vi "BrowseData.vi"(8 "ErrorIn(No Error)":errorcluster caption="entrée d'erreur (pas d'erreur)", 9 "MainProgQEvent":refnum<user-event>, 10 "MainProgQ":refnum<queue>, 11 "Interface en entrée":refnum<class "Interface.lvclass"> caption="DNL_LabVIEW Object in") -> (0 "sortie d'erreur":errorcluster, 3 "Interface en sortie":refnum<class "Interface.lvclass"> caption="DNL_LabVIEW Object out")   [LabVIEW 2019, in "Interface.lvclass"]
uses:
  Interface.lvclass
  BrowseDataStates.ctl
  ScanParams.ctl
  Interface.lvclass/Interface.ctl
panel:
  out "Header path":path
  out "Data path":path
  in  "YPar Sel":bool
  in  "Open2D":bool
  in  "Y Parameters":u16(ring) items=["AttoX.ReqPosition(um)", "AttoX.DetPos(um)", "AttoY.ReqPosition(um)", "AttoY.DetPos(um)", "MH150.Counts Ch1(ph)", "MH150.Counts Ch2(ph)", "MH150.Counts Chs Sum(ph)"]
  out "FilesPath":path[](array[path])
  out "Header String":string
  in  "CloseTreeStatus":bool
  in  "CloseTree":bool
  out "RangeString":string="??????"
  in  "Recheck Files":bool
  out "DateString":string="??????"
  in  "KeyWordFlt":bool
  in  "IncludeSubF":bool caption="Include SubFolders"
  in  "VarparFlt":bool
  in  "VarParam":string caption="Main Scan Parameter"
  in  "KeyWord":string
  in  "SessionFilt":bool
  in  "RangeFlt":bool
  in  "YearFlt":bool
  in  "DayFlt":bool
  in  "MonthFlt":bool
  in  "End Date":dbl=3629145600.0 format="%<%y/%m/%d>T"
  in  "Start Date":dbl format="%<%y/%m/%d>T"
  in  "Day":u8=1 min=1 max=31 step=1
  in  "Month":u8=1 min=1 max=12 step=1
  in  "Year":u16=2018 min=1960 max=2050 step=1
  in  "Session #":i32 min=0 max=1000 step=1
  out "VarPar":string
  out "CurveName":string
  in  "OpenCurve":bool
  in  "XPar Sel":bool
  in  "Data Folder Path":path
  in  "X Parameters":u16(ring) items=["AttoX.ReqPosition(um)", "AttoX.DetPos(um)", "AttoY.ReqPosition(um)", "AttoY.DetPos(um)", "MH150.Counts Ch1(ph)", "MH150.Counts Ch2(ph)", "MH150.Counts Chs Sum(ph)"]
  out "Curve Preview":cluster{"X Array":dbl[], "Y Array":dbl[]}(graph)
  out "DataPrev":string[][](array[string]) caption="File's Data Preview"
  in  "Arbre":string(tree)
  in  "stop":bool
  # "Filters"
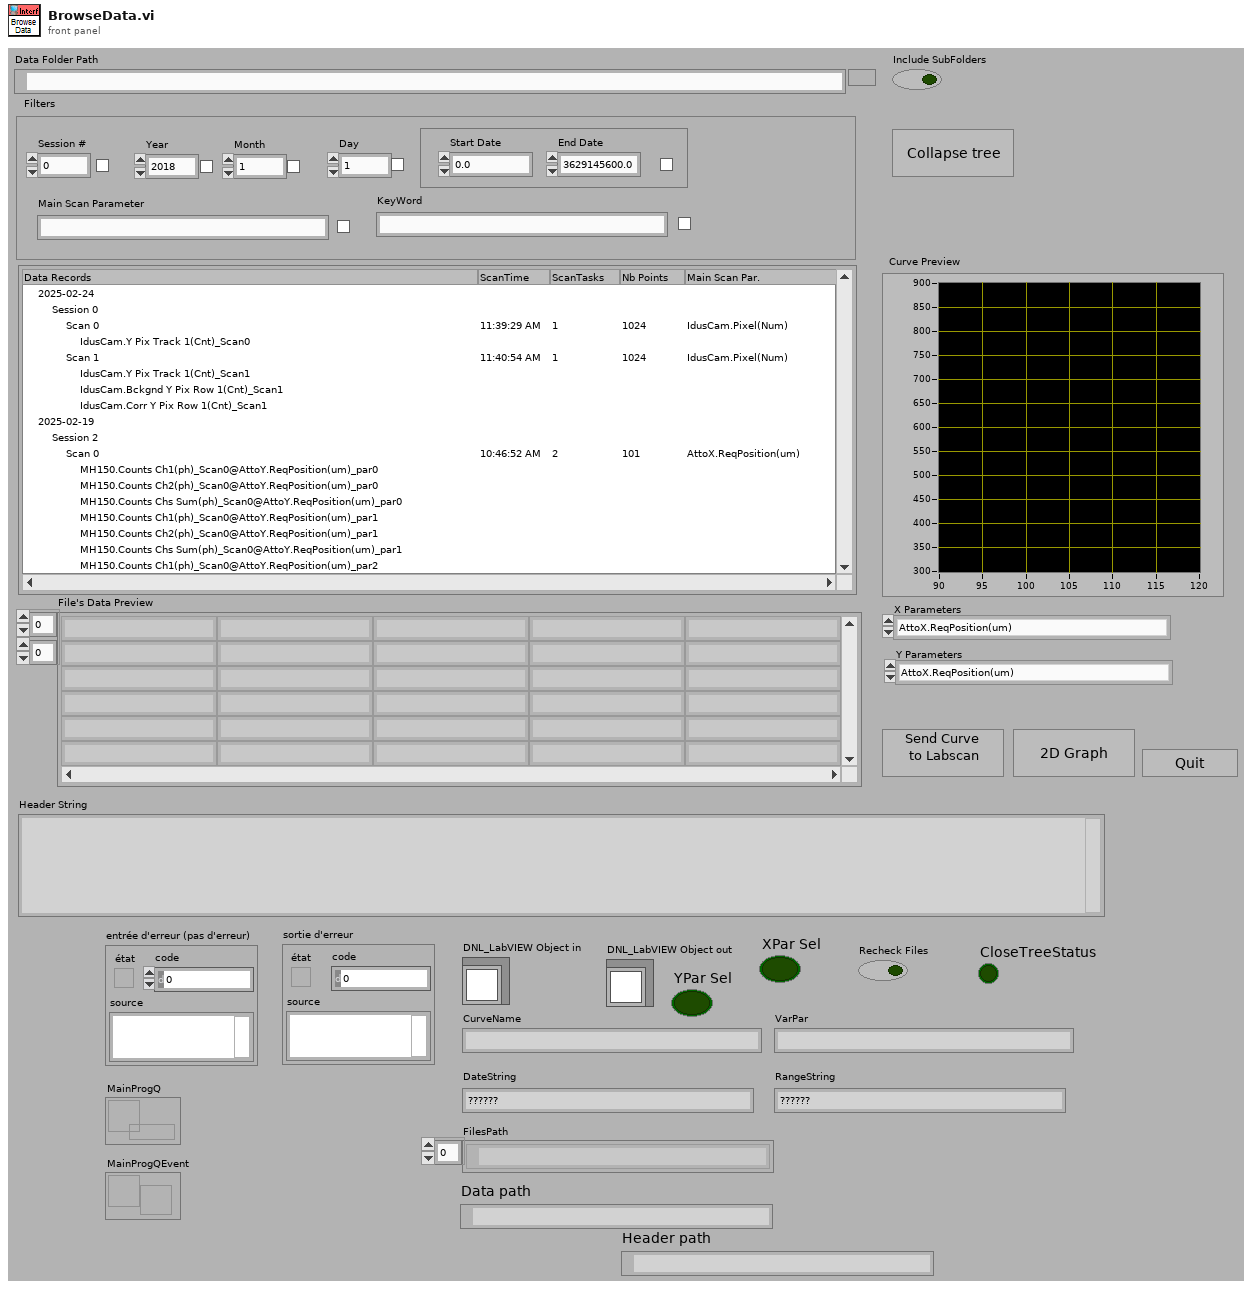
[diagram p1: front panel]
types:
  T1 = typedef "Interface.lvclass/ScanParams.ctl" = cluster{"Entête":string, "Scan list":string[], "NbCourbe":i32, "IndCourbe":i64, "NomDon":string[], "Session ":i32, "Date":string, "Time":string, "VarParams":string[][], "UserName":string, "ScanTableSize":i32[], "VarPar list":string[], "DescKeyword":string}
  T2 = typedef "BrowseDataStates.ctl" = enum16{"InitProg", "Delete File", "Opentxt", "LoadTree", "GetCurveData", "OpenCurve", "Open2D", "Stop"}
  T3 = enum8{"Enabled", "Disabled", "Disabled and Grayed Out"}
  T4 = enum16{"Enable", "Disable", "DisAndGrayed", "ReinitToDefVal", "EnumElementsArr"}
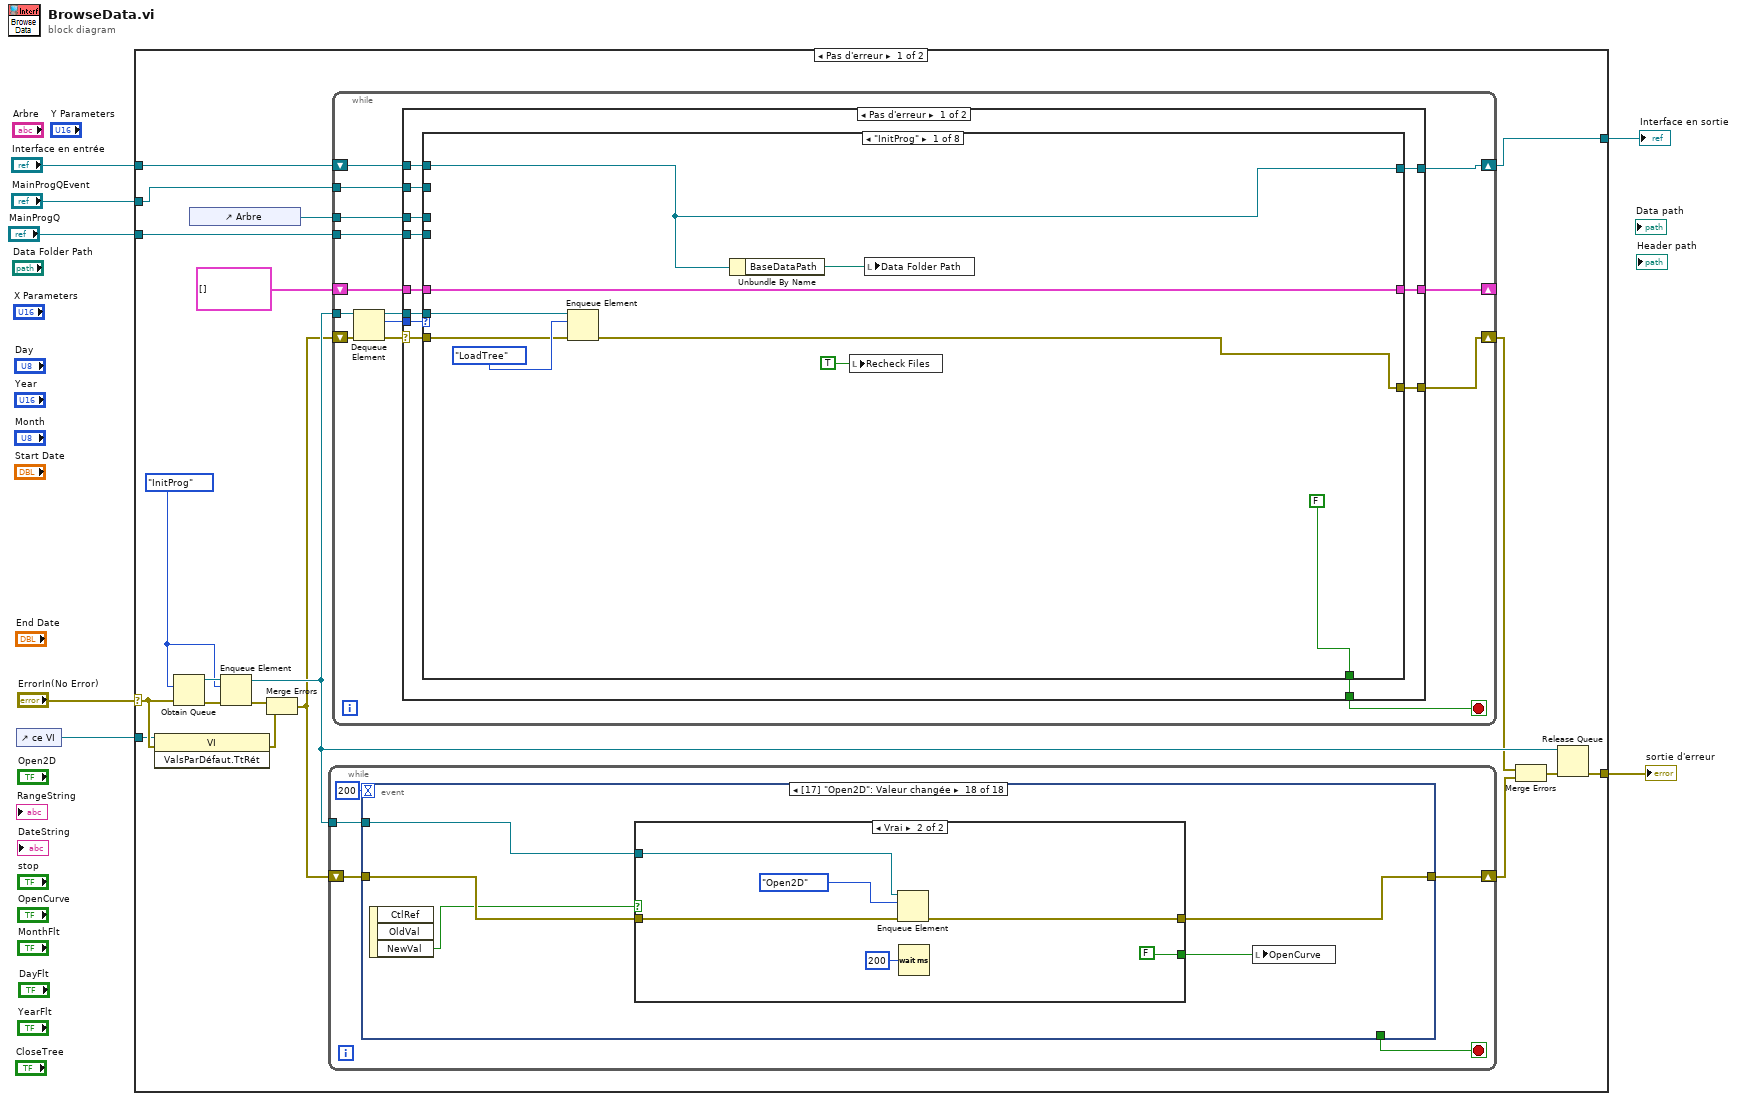
[diagram p0: block diagram]
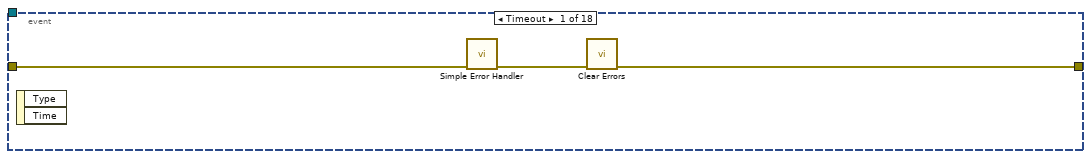
[diagram p2: hidden frame]
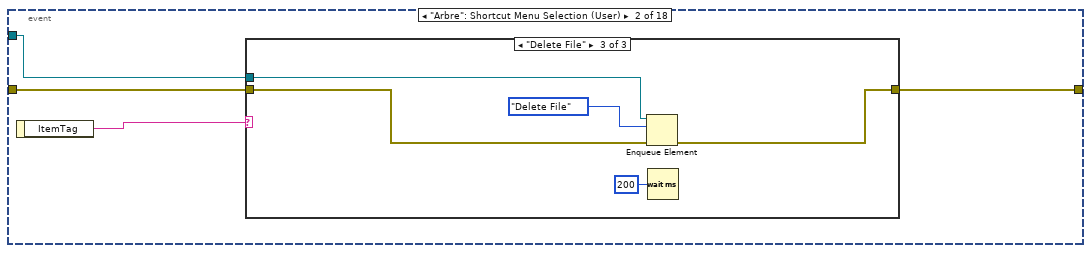
[diagram p3: hidden frame]
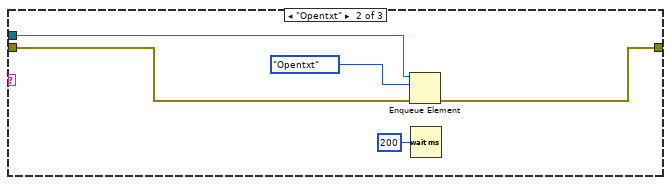
[diagram p5: hidden frame]
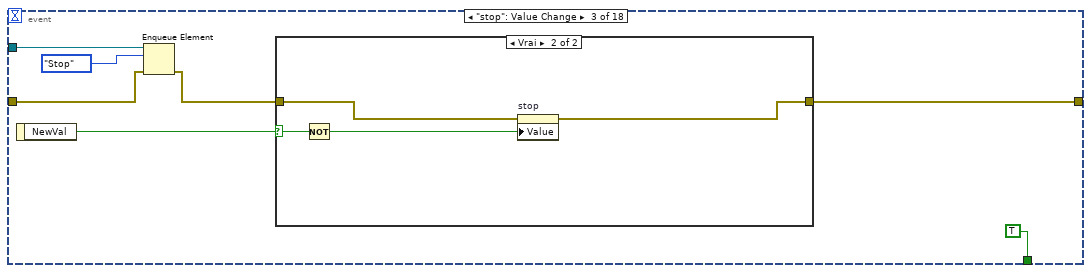
[diagram p6: hidden frame]
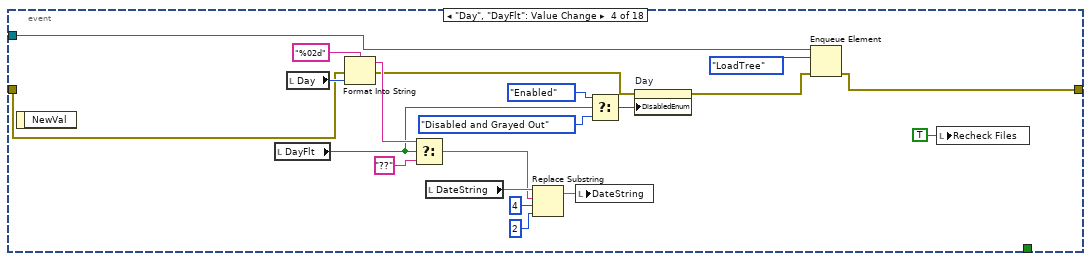
[diagram p8: hidden frame]
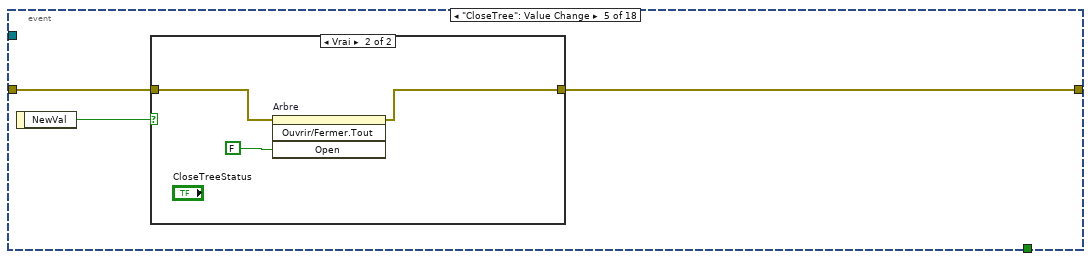
[diagram p9: hidden frame]
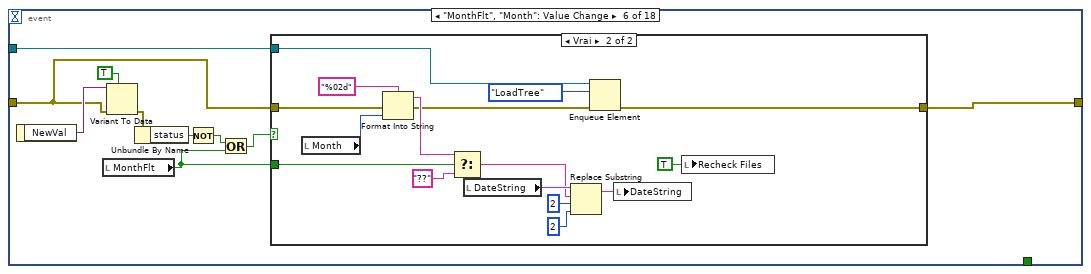
[diagram p11: hidden frame]
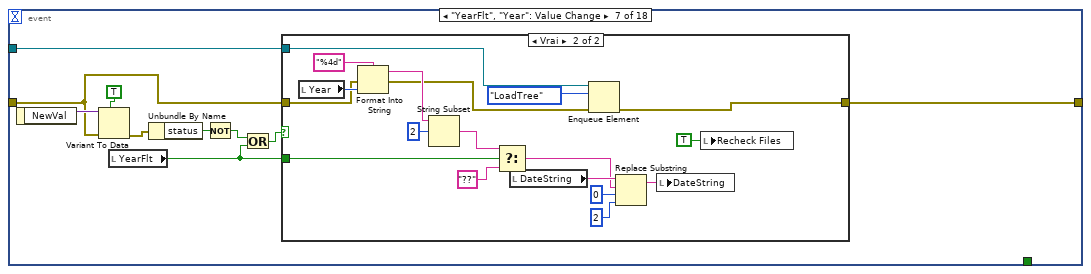
[diagram p13: hidden frame]
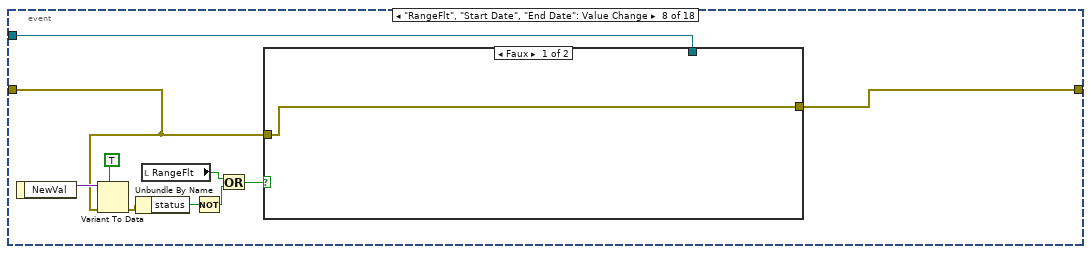
[diagram p15: hidden frame]
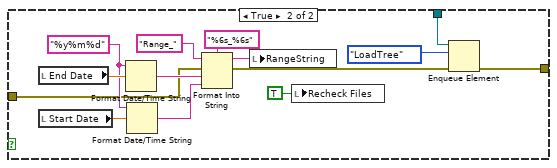
[diagram p16: hidden frame]
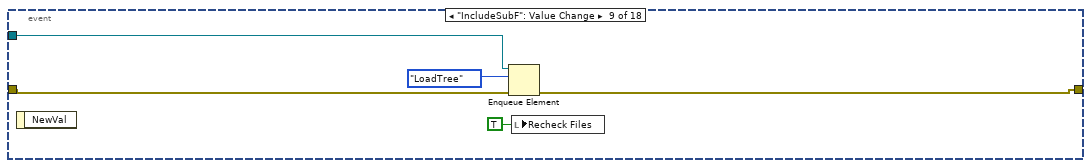
[diagram p17: hidden frame]
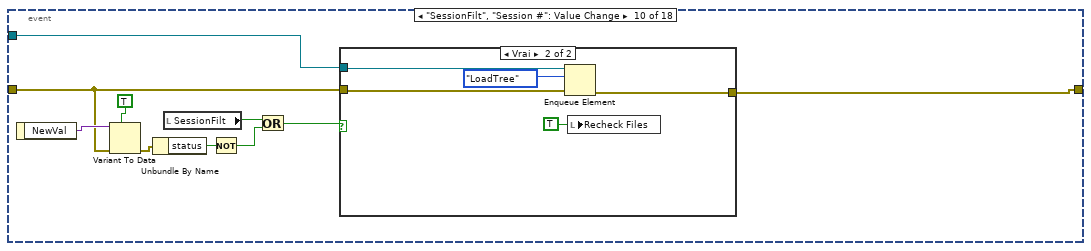
[diagram p18: hidden frame]
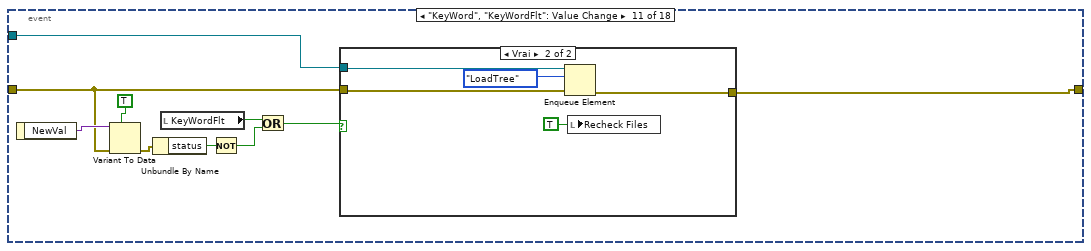
[diagram p20: hidden frame]
diagram:
  n1 = control-ref of="ce VI"() -> (w3:refnum<vi>)
  n2 = case shown="Pas d'erreur" "ErrorIn(No Error)" {
    selector: "ErrorIn(No Error)" -> [w13 w657]
    tunnel: [w23 w657] -> w6
    tunnel: "Interface en entrée" -> [w20 w656]
    tunnel: [w19 w656] -> w4
    tunnel: w3 -> [w12 _]
    tunnel: "MainProgQ" -> [w8 _]
    tunnel: "MainProgQEvent" -> [w9 _]
    frame No Error {
      w24 = BrowseDataStates."InitProg" ("Énum")
      n3 = invoke class="VI" method="ValsParDéfaut.TtRét"(reference=w12, error in=w13) -> (error out=w10:errorcluster)  [unwired: 1 in, 2 out]
      n4 = Obtain Queue(element data type=w24, error in (no error)=w13) -> (queue out=w25:refnum<queue>, error out=w26:errorcluster)  [unwired: 3 in, 1 out]
      n5 = control-ref of="Arbre"() -> (w18:refnum<vi>)
      n6 = Enqueue Element(queue=w25, element=w24, error in (no error)=w26) -> (queue out=w21:refnum<queue>, error out=w22:errorcluster)  [unwired: 1 in, 1 out]
      n7 = Merge Errors(w22, w10) -> (w11:errorcluster)
      n8 = while {
        shift-right: [w28] -> w15
        shift-left: w11 -> [w29]
        tunnel: w21 -> [w30]
        stop <- w27 stop-if-true
        n9 = event shown="[17] \"Open2D\": Valeur changée" {
          selector: _ -> [_ _ _ _ _ _ _ _ _ _ _ _ _ _ _ _ _ _]
          dyn-events: _ -> [_ _ _ _ _ _ _ _ _ _ _ _ _ _ _ _ _ _]
          timeout: 200 -> [_ _ _ _ _ _ _ _ _ _ _ _ _ _ _ _ _ _]
          tunnel: w30 -> [_ w35 w52 w63 _ w97 w124 w153 w170 w183 w199 w215 w224 w243 w256 _ w267 w280]
          tunnel: w29 -> [w34 w37 w54 w71 w83 w91 w121 w150 w172 w177 w193 w209 w229 w242 w253 w261 w266 w279]
          tunnel: [w32 w36 w55 w62 w82 w98 w125 w154 w171 w184 w200 w216 w225 w241 w257 w260 w268 w281] -> w28
          tunnel: [_ _ TRUE _ _ _ _ _ _ _ _ _ _ _ _ _ _ _] -> w27
          event Timeout {
            n10 = event-data() -> ()  [unwired: 1 in, 2 out]
            n11 = call <vilib>:"Simple Error Handler.vi"("error in (no error)"=w34) -> ("error out"=w33:errorcluster)  [unwired: 4 in, 4 out]
            n12 = call <vilib>:"Clear Errors.vi"("error in (no error)"=w33) -> ("error out"=w32:errorcluster)  [unwired: 5 in, 1 out]
          }
          event "Arbre": Shortcut Menu Selection (User) {
            n13 = event-data() -> ("ItemTag"=w38:string)  [unwired: 1 in]
            n14 = case shown="\"Delete File\"" w38 {
              tunnel: w37 -> [w39 w42 w47]
              tunnel: [w39 w41 w46] -> w36
              tunnel: w35 -> [_ w40 w45]
              frame Default {
              }
              frame "Opentxt" {
                n15 = Enqueue Element(queue=w40, element=BrowseDataStates."Opentxt" ("Énum"), error in (no error)=w42) -> (error out=w41:errorcluster)  [unwired: 1 in, 2 out]
                n16 = Wait (ms)(milliseconds to wait=u32 200 ("attente (ms)")) -> ()  [unwired: 1 out]
              }
              frame "Delete File" {
                n17 = Enqueue Element(queue=w45, element=BrowseDataStates."Delete File" ("Énum"), error in (no error)=w47) -> (error out=w46:errorcluster)  [unwired: 1 in, 2 out]
                n18 = Wait (ms)(milliseconds to wait=u32 200 ("attente (ms)")) -> ()  [unwired: 1 out]
              }
            }
          }
          event "stop": Value Change {
            n19 = event-data() -> ("NewVal"=w56:bool)  [unwired: 1 in]
            n20 = Enqueue Element(queue=w52, element=BrowseDataStates."Stop" ("Énum"), error in (no error)=w54) -> (error out=w53:errorcluster)  [unwired: 1 in, 2 out]
            n21 = case shown="Vrai" w56 {
              selector: w56 -> [_ w61]
              tunnel: w53 -> [w57 w59]
              tunnel: [w57 w58] -> w55
              frame False {
              }
              frame True {
                n22 = Not(x=w61) -> (.not. x?=w60:bool)
                n23 = property on="stop" class="Bool (strict)"(error in=w59, "Value"=w60) -> (error out=w58:errorcluster)  [unwired: 1 in, 1 out]
              }
            }
          }
          event "Day", "DayFlt": Value Change {
            n24 = event-data() -> ()  [unwired: 1 in, 1 out]
            n25 = local read "DayFlt"() -> (w70:bool)
            n26 = local read "Day"() -> (w79:u8)
            n27 = Format Into String(format string="%02d" ("chaîne de format"), error in=w71, w79) -> (resulting string=w74:string, error out=w67:errorcluster)  [unwired: 1 in]
            n28 = Select(t=w74, s=w70, f="??" ("cas faux")) -> (s? t:f=w73:string)
            n29 = local read "DateString"() -> (w80:string)
            n30 = Replace Substring(2:2 ("longueur (long. de la sous-chaîne)"), 3:4 ("offset (0)"), 4:w73, 5:w80) -> (1:w75:string)  [unwired: 1 out]
            n31 = local write "DateString"(w75) -> ()
            n32 = Select(t=T3."Enabled" ("Désactivé"), s=w70, f=T3."Disabled and Grayed Out" ("Désactivé")) -> (s? t:f=w66:T3)
            n33 = property on="Day" class="NumNb (strict)"(error in=w67, "DisabledEnum"=w66) -> (error out=w64:errorcluster)  [unwired: 1 in, 1 out]
            n34 = Enqueue Element(queue=w63, element=BrowseDataStates."LoadTree" ("Énum"), error in (no error)=w64) -> (error out=w62:errorcluster)  [unwired: 1 in, 2 out]
            n35 = local write "Recheck Files"(TRUE ("Recheck Files")) -> ()
          }
          event "CloseTree": Value Change {
            n36 = event-data() -> ("NewVal"=w84:bool)  [unwired: 1 in]
            n37 = case shown="Vrai" w84 {
              tunnel: w83 -> [w85 w88]
              tunnel: [w85 w87] -> w82
              frame False {
              }
              frame True {
                n38 = invoke on="Arbre" class="Arbre (strict)" method="Ouvrir/Fermer.Tout"(error in=w88, "Open"=FALSE ("Ouvrir ?")) -> (error out=w87:errorcluster)  [unwired: 2 in, 3 out]
              }
            }
          }
          event "MonthFlt", "Month": Value Change {
            n39 = event-data() -> ("NewVal"=w95:variant)  [unwired: 1 in]
            n40 = local read "MonthFlt"() -> (w89:bool)
            n41 = Variant To Data(error in=w91, type=TRUE, Variant=w95) -> (error out=w90:errorcluster)  [unwired: 1 out]
            n42 = Unbundle By Name(w90) -> ("status"=w94:bool)
            n43 = Not(x=w94) -> (.not. x?=w93:bool)
            n44 = Or(x=w93, y=w89) -> (x .or. y?=w92:bool)
            n45 = case shown="Vrai" w92 {
              tunnel: [w99 w104] -> w98
              tunnel: w97 -> [_ w103]
              tunnel: w91 -> [w99 w102]
              tunnel: w89 -> [_ w101]
              frame False {
              }
              frame True {
                n46 = local read "Month"() -> (w113:u8)
                n47 = Format Into String(format string="%02d" ("chaîne de format"), error in=w102, w113) -> (resulting string=w108:string, error out=w100:errorcluster)  [unwired: 1 in]
                n48 = Select(t=w108, s=w101, f="??" ("cas faux")) -> (s? t:f=w107:string)
                n49 = local read "DateString"() -> (w114:string)
                n50 = Replace Substring(2:2 ("longueur (long. de la sous-chaîne)"), 3:2 ("offset (0)"), 4:w107, 5:w114) -> (1:w109:string)  [unwired: 1 out]
                n51 = Enqueue Element(queue=w103, element=BrowseDataStates."LoadTree" ("Énum"), error in (no error)=w100) -> (error out=w104:errorcluster)  [unwired: 1 in, 2 out]
                n52 = local write "DateString"(w109) -> ()
                n53 = local write "Recheck Files"(TRUE ("Recheck Files")) -> ()
              }
            }
          }
          event "YearFlt", "Year": Value Change {
            n54 = event-data() -> ("NewVal"=w123:variant)  [unwired: 1 in]
            n55 = Variant To Data(error in=w121, type=TRUE, Variant=w123) -> (error out=w120:errorcluster)  [unwired: 1 out]
            n56 = local read "YearFlt"() -> (w116:bool)
            n57 = Unbundle By Name(w120) -> ("status"=w119:bool)
            n58 = Not(x=w119) -> (.not. x?=w117:bool)
            n59 = Or(x=w117, y=w116) -> (x .or. y?=w118:bool)
            n60 = case shown="Vrai" w118 {
              tunnel: w121 -> [w126 w135]
              tunnel: w116 -> [_ w134]
              tunnel: [w126 w132] -> w125
              tunnel: w124 -> [_ w131]
              frame False {
              }
              frame True {
                n61 = local read "Year"() -> (w142:u16)
                n62 = Format Into String(format string="%4d" ("chaîne de format"), error in=w135, w142) -> (resulting string=w130:string, error out=w127:errorcluster)  [unwired: 1 in]
                n63 = String Subset(string=w130, offset (0)=2) -> (substring=w128:string)  [unwired: 1 in]
                n64 = Select(t=w128, s=w134, f="??" ("cas faux")) -> (s? t:f=w137:string)
                n65 = local read "DateString"() -> (w143:string)
                n66 = Enqueue Element(queue=w131, element=BrowseDataStates."LoadTree" ("Énum"), error in (no error)=w127) -> (error out=w132:errorcluster)  [unwired: 1 in, 2 out]
                n67 = Replace Substring(2:2 ("longueur (long. de la sous-chaîne)"), 3:0 ("offset (0)"), 4:w137, 5:w143) -> (1:w138:string)  [unwired: 1 out]
                n68 = local write "DateString"(w138) -> ()
                n69 = local write "Recheck Files"(TRUE ("Recheck Files")) -> ()
              }
            }
          }
          event "RangeFlt", "Start Date", "End Date": Value Change {
            n70 = event-data() -> ("NewVal"=w152:variant)  [unwired: 1 in]
            n71 = Variant To Data(error in=w150, type=TRUE, Variant=w152) -> (error out=w149:errorcluster)  [unwired: 1 out]
            n72 = Unbundle By Name(w149) -> ("status"=w148:bool)
            n73 = local read "RangeFlt"() -> (w146:bool)
            n74 = Not(x=w148) -> (.not. x?=w147:bool)
            n75 = Or(x=w146, y=w147) -> (x .or. y?=w145:bool)
            n76 = case shown="Faux" w145 {
              tunnel: [w155 w166] -> w154
              tunnel: w153 -> [_ w165]
              tunnel: w150 -> [w155 w156]
              frame False {
              }
              frame True {
                w162 = "%y%m%d" ("chaîne de format de l'heure (%c)")
                n77 = local read "End Date"() -> (w164:dbl)
                n78 = local read "Start Date"() -> (w163:dbl)
                n79 = Format Date/Time String(time format string (%c)=w162, seconds (now)=w164) -> (date/time string=w160:string)  [unwired: 1 in]
                n80 = Format Date/Time String(time format string (%c)=w162, seconds (now)=w163) -> (date/time string=w161:string)  [unwired: 1 in]
                n81 = Format Into String(format string="%6s_%6s" ("chaîne de format"), initial string="Range_" ("chaîne initiale"), error in=w156, w160, w161) -> (resulting string=w158:string, error out=w157:errorcluster)
                n82 = local write "RangeString"(w158) -> ()
                n83 = local write "Recheck Files"(TRUE ("Recheck Files")) -> ()
                n84 = Enqueue Element(queue=w165, element=BrowseDataStates."LoadTree" ("Énum"), error in (no error)=w157) -> (error out=w166:errorcluster)  [unwired: 1 in, 2 out]
              }
            }
          }
          event "IncludeSubF": Value Change {
            n85 = event-data() -> ()  [unwired: 1 in, 1 out]
            n86 = Enqueue Element(queue=w170, element=BrowseDataStates."LoadTree" ("Énum"), error in (no error)=w172) -> (error out=w171:errorcluster)  [unwired: 1 in, 2 out]
            n87 = local write "Recheck Files"(TRUE ("Recheck Files")) -> ()
          }
          event "SessionFilt", "Session #": Value Change {
            n88 = event-data() -> ("NewVal"=w178:variant)  [unwired: 1 in]
            n89 = Variant To Data(error in=w177, type=TRUE, Variant=w178) -> (error out=w181:errorcluster)  [unwired: 1 out]
            n90 = Unbundle By Name(w181) -> ("status"=w180:bool)
            n91 = local read "SessionFilt"() -> (w175:bool)
            n92 = Not(x=w180) -> (.not. x?=w179:bool)
            n93 = Or(x=w175, y=w179) -> (x .or. y?=w176:bool)
            n94 = case shown="Vrai" w176 {
              tunnel: [w185 w188] -> w184
              tunnel: w183 -> [_ w187]
              tunnel: w177 -> [w185 w186]
              frame False {
              }
              frame True {
                n95 = Enqueue Element(queue=w187, element=BrowseDataStates."LoadTree" ("Énum"), error in (no error)=w186) -> (error out=w188:errorcluster)  [unwired: 1 in, 2 out]
                n96 = local write "Recheck Files"(TRUE ("Recheck Files")) -> ()
              }
            }
          }
          event "KeyWord", "KeyWordFlt": Value Change {
            n97 = event-data() -> ("NewVal"=w194:variant)  [unwired: 1 in]
            n98 = Variant To Data(error in=w193, type=TRUE, Variant=w194) -> (error out=w197:errorcluster)  [unwired: 1 out]
            n99 = Unbundle By Name(w197) -> ("status"=w196:bool)
            n100 = local read "KeyWordFlt"() -> (w191:bool)
            n101 = Not(x=w196) -> (.not. x?=w195:bool)
            n102 = Or(x=w191, y=w195) -> (x .or. y?=w192:bool)
            n103 = case shown="Vrai" w192 {
              tunnel: [w201 w204] -> w200
              tunnel: w199 -> [_ w203]
              tunnel: w193 -> [w201 w202]
              frame False {
              }
              frame True {
                n104 = Enqueue Element(queue=w203, element=BrowseDataStates."LoadTree" ("Énum"), error in (no error)=w202) -> (error out=w204:errorcluster)  [unwired: 1 in, 2 out]
                n105 = local write "Recheck Files"(TRUE ("Recheck Files")) -> ()
              }
            }
          }
          event "VarparFlt", "VarParam": Value Change {
            n106 = event-data() -> ("NewVal"=w210:variant)  [unwired: 1 in]
            n107 = Variant To Data(error in=w209, type=TRUE, Variant=w210) -> (error out=w213:errorcluster)  [unwired: 1 out]
            n108 = Unbundle By Name(w213) -> ("status"=w212:bool)
            n109 = local read "VarparFlt"() -> (w207:bool)
            n110 = Not(x=w212) -> (.not. x?=w211:bool)
            n111 = Or(x=w207, y=w211) -> (x .or. y?=w208:bool)
            n112 = case shown="Vrai" w208 {
              tunnel: [w217 w220] -> w216
              tunnel: w215 -> [_ w219]
              tunnel: w209 -> [w217 w218]
              frame False {
              }
              frame True {
                n113 = Enqueue Element(queue=w219, element=BrowseDataStates."LoadTree" ("Énum"), error in (no error)=w218) -> (error out=w220:errorcluster)  [unwired: 1 in, 2 out]
                n114 = local write "Recheck Files"(TRUE ("Recheck Files")) -> ()
              }
            }
          }
          event "Arbre": Value Change {
            n115 = event-data() -> ("CtlRef"=w231:refnum<vi>, "NewVal"=w230:string)  [unwired: 1 in]
            n116 = property class="Arbre (strict)"(reference=w231, error in=w229, "Active Item Tag"=w230) -> (error out=w226:errorcluster, "Indent Level"=w223:i32)  [unwired: 1 out]
            n117 = Equal?(x=w223, y=3 ("x")) -> (x = y?=w227:bool)
            n118 = case shown="Vrai" w227 {
              tunnel: w226 -> [w232 w240]
              tunnel: [w232 w239] -> w225
              tunnel: w224 -> [_ w238]
              tunnel: w223 -> [w235 _]
              frame False {
                n119 = Equal?(x=w235, y=2) -> (x = y?=w233:bool)
                n120 = case shown="Vrai" w233 {
                  frame False {
                  }
                  frame True {
                  }
                }
              }
              frame True {
                w236 = FALSE ("XPar Sel")
                n121 = local write "XPar Sel"(w236) -> ()
                n122 = local write "YPar Sel"(w236) -> ()
                n123 = Enqueue Element(queue=w238, element=BrowseDataStates."GetCurveData" ("Énum"), error in (no error)=w240) -> (error out=w239:errorcluster)  [unwired: 1 in, 2 out]
              }
            }
          }
          event "Data Folder Path": Value Change {
            n124 = event-data() -> ("OldVal"=w246:path, "NewVal"=w245:path)  [unwired: 1 in, 1 out]
            n125 = Not Equal?(x=w246, y=w245) -> (x != y?=w244:bool)
            n126 = case shown="Vrai" w244 {
              tunnel: w243 -> [_ w251]
              tunnel: w242 -> [w247 w250]
              tunnel: [w247 w249] -> w241
              frame False {
              }
              frame True {
                n127 = Enqueue Element(queue=w251, element=BrowseDataStates."LoadTree" ("Énum"), error in (no error)=w250) -> (error out=w249:errorcluster)  [unwired: 1 in, 2 out]
                n128 = local write "Recheck Files"(TRUE ("Recheck Files")) -> ()
              }
            }
          }
          event "X Parameters": Value Change {
            n129 = event-data() -> ()  [unwired: 1 in, 3 out]
            n130 = flat-sequence {
              tunnel: [w258] -> w254
              tunnel: w253 -> [w258]
              frame #0 {
                n131 = local write "XPar Sel"(TRUE ("XPar Sel")) -> ()
              }
            }
            n132 = Enqueue Element(queue=w256, element=BrowseDataStates."GetCurveData" ("Énum"), error in (no error)=w254) -> (error out=w257:errorcluster)  [unwired: 1 in, 2 out]
          }
          event "Y Parameters": Value Change {
            n133 = event-data() -> ()  [unwired: 1 in, 3 out]
            n134 = flat-sequence {
              tunnel: [w262] -> w260
              tunnel: w261 -> [w262]
              frame #0 {
                n135 = local write "YPar Sel"(TRUE ("XPar Sel")) -> ()
              }
            }
          }
          event "OpenCurve": Value Change {
            n136 = event-data() -> ("NewVal"=w265:bool)  [unwired: 1 in, 2 out]
            n137 = case shown="Vrai" w265 {
              tunnel: [w269 w276] -> w268
              tunnel: w267 -> [_ w275]
              tunnel: w266 -> [w269 w274]
              tunnel: [FALSE ("OpenCurve") FALSE ("OpenCurve")] -> w264
              frame False {
              }
              frame True {
                n138 = Enqueue Element(queue=w275, element=BrowseDataStates."OpenCurve" ("Énum"), error in (no error)=w274) -> (error out=w276:errorcluster)  [unwired: 1 in, 2 out]
                n139 = Wait (ms)(milliseconds to wait=u32 200 ("attente (ms)")) -> ()  [unwired: 1 out]
              }
            }
            n140 = local write "OpenCurve"(w264) -> ()
          }
          event "Open2D": Value Change {
            n141 = event-data() -> ("NewVal"=w278:bool)  [unwired: 1 in, 2 out]
            n142 = case shown="Vrai" w278 {
              tunnel: [w282 w289] -> w281
              tunnel: w280 -> [_ w288]
              tunnel: w279 -> [w282 w287]
              tunnel: [FALSE ("OpenCurve") FALSE ("OpenCurve")] -> w277
              frame False {
              }
              frame True {
                n143 = Enqueue Element(queue=w288, element=BrowseDataStates."Open2D" ("Énum"), error in (no error)=w287) -> (error out=w289:errorcluster)  [unwired: 1 in, 2 out]
                n144 = Wait (ms)(milliseconds to wait=u32 200 ("attente (ms)")) -> ()  [unwired: 1 out]
              }
            }
            n145 = local write "OpenCurve"(w277) -> ()
          }
        }
      }
      n146 = while {
        tunnel: w21 -> [w301]
        shift-right: [w297] -> w16
        shift-left: w11 -> [w299]
        shift-right: [w296] -> w19
        shift-left: w20 -> [w295]
        tunnel: w18 -> [w294]
        shift-right: [w293] -> _
        shift-left: T1[] [] ("Headers") -> [w292]
        tunnel: w9 -> [w291]
        tunnel: w8 -> [w290]
        stop <- w298 stop-if-true
        n147 = Dequeue Element(queue=w301, error in (no error)=w299) -> (queue out=w300:refnum<queue>, element=w302:T2, error out=w303:errorcluster)  [unwired: 1 in, 1 out]
        n148 = case shown="Pas d'erreur" w303 {
          selector: w303 -> [w313 w654]
          tunnel: w302 -> [w315 _]
          tunnel: w300 -> [w314 _]
          tunnel: [w312 FALSE] -> w298
          tunnel: [w311 w651] -> w297
          tunnel: [w310 w653] -> w296
          tunnel: w295 -> [w309 w653]
          tunnel: w294 -> [w308 _]
          tunnel: [w307 w652] -> w293
          tunnel: w292 -> [w306 w652]
          tunnel: w291 -> [w305 _]
          tunnel: w290 -> [w304 _]
          frame No Error {
            n149 = case shown="\"InitProg\"" w315 {
              tunnel: w314 -> [w321 _ _ _ w523 _ _ _]
              tunnel: w313 -> [w318 w337 w394 w500 w550 w597 w639 w649]
              tunnel: [FALSE FALSE _ _ _ _ _ TRUE] -> w312
              tunnel: [w316 w330 w390 w475 w524 w582 w609 w649] -> w311
              tunnel: [w323 w360 w385 w496 w546 w584 w641 w647] -> w310
              tunnel: w309 -> [w323 w360 w385 w496 w546 w598 w642 w647]
              tunnel: w308 -> [_ w359 w395 w501 w551 _ _ _]
              tunnel: [w319 w358 w387 w497 w547 w596 w646 w648] -> w307
              tunnel: w306 -> [w319 w343 w387 w497 w547 w596 w646 w648]
              tunnel: w305 -> [_ _ _ _ _ w586 _ _]
              tunnel: w304 -> [_ _ _ _ _ w585 _ _]
              frame "InitProg" {
                n150 = Enqueue Element(queue=w321, element=BrowseDataStates."LoadTree" ("Énum"), error in (no error)=w318) -> (error out=w316:errorcluster)  [unwired: 1 in, 2 out]
                n151 = Unbundle By Name(w323) -> ("BaseDataPath"=w322:path)
                n152 = local write "Recheck Files"(TRUE ("Recheck Files")) -> ()
                n153 = local write "Data Folder Path"(w322) -> ()
              }
              frame "LoadTree" {
                n154 = control-ref of="This VI"() -> (w336:refnum<vi>)
                n155 = property class="VI"(reference=w336, error in=w337) -> (error out=w335:errorcluster, "Panel"=w334:refnum<vi>)  [unwired: 1 out]
                n156 = property class="FA"(reference=w334, error in=w335, "DeferPanUpdts"=TRUE ("Defer Panel Updates")) -> (reference out=w333:refnum<vi>, error out=w328:errorcluster)
                n157 = local read "RangeString"() -> (w339:string)
                n158 = local read "DateString"() -> (w340:string)
                n159 = Select(t="Session #", s="SessionFilt", f=-1 ("cas faux")) -> (s? t:f=w344:i32)
                n160 = Select(t="VarParam", s="VarparFlt", f="" ("cas faux")) -> (s? t:f=w348:string)
                n161 = call <vilib>:"Set Busy.vi"("error in (no error)"=w328) -> ("error out"=w327:errorcluster)  [unwired: 9 in, 1 out]
                n162 = local read "Data Folder Path"() -> (w357:path)
                n163 = Select(t="KeyWord", s="KeyWordFlt", f="" ("cas faux")) -> (s? t:f=w352:string)
                n164 = Select(t=w339, s="RangeFlt", f=w340) -> (s? t:f=w338:string)
                n165 = call "DataTree_LS1.vi"("Arbre"=w359, "Data Folder Path"=w357, "ScanParamsIn"=w343, "VarParam"=w348, "Date String"=w338, "Session"=w344, "error in (no err)"=w327, "IncludeSubF"="IncludeSubF", "Recheck Files"="Recheck Files", "KeyWord"=w352) -> ("Headers Out"=w358:T1[], "FilesPath"=→"FilesPath":path[], "error out"=w326:errorcluster)  [unwired: 1 in, 2 out]
                n166 = call <vilib>:"Unset Busy.vi"("error in (no error)"=w326) -> ("error out"=w325:errorcluster)  [unwired: 10 in]
                n167 = property class="FA"(reference=w333, error in=w325, "DeferPanUpdts"=FALSE ("Defer Panel Updates")) -> (error out=w330:errorcluster)  [unwired: 1 out]
              }
              frame "GetCurveData" {
                n168 = property class="Arbre (strict)"(reference=w395, error in=w394) -> (error out=w379:errorcluster, "Active Item Tag"=w378:string)  [unwired: 1 out]
                n169 = Scan From String(format string="%4s-%2s-%2s_S%d_Sc%d_%d_f%d" ("chaîne de format"), input string=w378, error in=w379, default 5=i64 0 ("valeur par défaut 5")) -> (error out=w380:errorcluster, output 6=w381:i32, output 7=w383:i32)  [unwired: 12 in, 2 out]
                n170 = case shown="Pas d'erreur" w380 {
                  selector: w380 -> [w396 _]
                  tunnel: w383 -> [w398 _]
                  tunnel: [w398 w400] -> w363
                  tunnel: [w397 w399] -> w382
                  tunnel: w381 -> [w397 _]
                  tunnel: [w396 w401] -> w372
                  tunnel: w379 -> [_ w402]
                  tunnel: w378 -> [_ w405]
                  tunnel: "%4s-%2s-%2s_S%d_Sc%d_%d_%d_f%d" ("chaîne de format") -> [_ w404]
                  frame No Error {
                  }
                  frame Error {
                    n171 = Scan From String(format string=w404, input string=w405, error in=w402, default 5=i64 0 ("valeur par défaut 5")) -> (error out=w401:errorcluster, output 7=w399:i32, output 8=w400:i32)  [unwired: 14 in, 2 out]
                  }
                }
                n172 = local read "FilesPath"() -> (w384:path[])
                n173 = Index Array(array=w384, index=w363) -> (element=w376:path)
                n174 = Strip Path(path=w376) -> (stripped path=w366:path, name=w375:string)
                n175 = Search and Replace String(input string=w375, search string="Header" ("sous-chaîne (\"\")"), replace string="Data" ("chaîne de remplacement (\"\")"), error in=w372) -> (result string=w370:string, error out=w371:errorcluster)  [unwired: 4 in, 2 out]
                n176 = Search and Replace String(input string=w370, search string=".dat" ("chaîne recherchée"), replace string=".txt" ("chaîne de remplacement (\"\")"), error in=w371) -> (result string=w367:string, error out=w364:errorcluster)  [unwired: 4 in, 2 out]
                n177 = case shown="Faux" "XPar Sel" {
                  tunnel: [w417 w454] -> w391
                  tunnel: w364 -> [w416 w455]
                  tunnel: [w415 w453] -> w389
                  tunnel: [w412 TRUE] -> w388
                  tunnel: w387 -> [w411 _]
                  tunnel: w363 -> [w410 _]
                  tunnel: "YPar Sel" -> [w406 _]
                  frame False {
                    w408 = 0 ("indice (ligne)")
                    # "Get row of main var par"
                    n178 = Index Array(array=w411, index=w410) -> (element=w418:T1)
                    n179 = Unbundle By Name(w418) -> ("NomDon"=w407:string[], "VarParams"=w409:string[][])
                    n180 = case shown="Faux" w406 {
                      tunnel: w409 -> [w430 _]
                      tunnel: w408 -> [w427 _]
                      tunnel: w407 -> [w424 _]
                      frame False {
                        n181 = control-ref of="Open2D"() -> (w422:refnum<vi>)
                        n182 = Index Array(array=w430, index (row)=1 ("indice désactivé (col)"), index (col)=w427) -> (element=w426:string)
                        n183 = Match Pattern(string=w426, regular expression="_" ("expression régulière")) -> (before substring=w425:string, offset past match=w423:i32)  [unwired: 1 in, 2 out]
                        n184 = case shown="0, Par défaut" w423 {
                          tunnel: w425 -> [w437 _]
                          tunnel: w424 -> [w432 _]
                          tunnel: w422 -> [w431 w443]
                          frame 0, Default {
                            n185 = for {
                              tunnel: w437 -> [w442]
                              tunnel: w432 -> [w439] mode=indexing
                              tunnel: [w441] -> w435
                              tunnel: [w438] -> w434
                              i -> [w441]
                              stop <- w438 stop-if-true
                              n186 = Match Pattern(string=w439, regular expression=w442) -> (offset past match=w440:i32)  [unwired: 1 in, 3 out]
                              n187 = Greater Or Equal To 0?(x=w440) -> (x >= 0?=w438:bool)
                            }
                            n188 = Select(t=w435, s=w434, f=0 ("cas faux")) -> (s? t:f=w433:i32)
                            n189 = property on="Y Parameters" class="MDér (strict)"("Strings []"=w432, "Value"=w433) -> ()  [unwired: 2 in, 2 out]
                            n190 = call <userlib>:"SetCtrlPropGenSgl.vi"("Controls"=w431) -> ()  [unwired: 5 in, 2 out]
                          }
                          frame -1 {
                            n191 = property on="Y Parameters" class="MDér (strict)"("Strings []"=string[] [] ("Chaînes []"), "Value"=0 ("indice (ligne)")) -> ()  [unwired: 2 in, 2 out]
                            n192 = call <userlib>:"SetCtrlPropGenSgl.vi"("Énum"=T4."DisAndGrayed", "Controls"=w443) -> ()  [unwired: 4 in, 2 out]
                          }
                        }
                      }
                      frame True {
                      }
                    }
                    n193 = Index Array(array=w409, index (row)=w408, index (col)=w408) -> (element=w421:string)
                    n194 = Match Pattern(string=w421, regular expression="_" ("expression régulière")) -> (before substring=w419:string)  [unwired: 1 in, 3 out]
                    n195 = for {
                      tunnel: w419 -> [w451]
                      tunnel: w407 -> [w448] mode=indexing
                      tunnel: [w450] -> w414
                      tunnel: [w447] -> w412
                      i -> [w450]
                      stop <- w447 stop-if-true
                      n196 = Match Pattern(string=w448, regular expression=w451) -> (offset past match=w449:i32)  [unwired: 1 in, 3 out]
                      n197 = Greater Or Equal To 0?(x=w449) -> (x >= 0?=w447:bool)
                    }
                    n198 = Select(t=w414, s=w412, f=0 ("cas faux")) -> (s? t:f=w415:i32)
                    n199 = property on="X Parameters" class="MDér (strict)"(error in=w416, "Strings []"=w407, "Value"=w415) -> (error out=w417:errorcluster)  [unwired: 1 in, 1 out]
                  }
                  frame True {
                    # "get  the selected x data row"
                    n200 = property on="X Parameters" class="MDér (strict)"(error in=w455) -> (error out=w454:errorcluster, "Value"=w453:u16)  [unwired: 1 in, 1 out]
                  }
                }
                n201 = Build Path(base path=w366, name or relative path=w367) -> (appended path=w365:path)
                n202 = case shown="Pas d'erreur" w364 {
                  tunnel: w376 -> [w457 _]
                  tunnel: w365 -> [w458 _]
                  tunnel: w391 -> [w466 w473]
                  tunnel: [w464 w471] -> w390
                  tunnel: w389 -> [w463 _]
                  tunnel: w382 -> [w462 _]
                  frame No Error {
                    n203 = local write "Header path"(w457) -> ()
                    n204 = local write "Data path"(w458) -> ()
                    n205 = call "DataReadTxt.vi"("Chemin Header"=w457, "chemin Data"=w458, "ScanlistIndex"=w462, "error in"=w466, "VarParIndex"=w463) -> ("Header String"=→"Header String":string, "VarPar"=→"VarPar":string, "Data Preview"=→"DataPrev":string[][], "X Array"=w468:dbl[], "Y Array"=w467:dbl[], "CurveName"=→"CurveName":string, "error out"=w464:errorcluster)  [unwired: 3 in, 1 out]
                    n206 = Bundle("X Array"=w468, "Y Array"=w467) -> (→"Curve Preview":cluster{"X Array":dbl[], "Y Array":dbl[]})  [unwired: 1 in]
                  }
                  frame Error {
                    n207 = call <vilib>:"Clear Errors.vi"("error in (no error)"=w473) -> ("error out"=w471:errorcluster)  [unwired: 5 in, 1 out]
                    n208 = local write "Data path"(path "" ("Data path")) -> ()
                    n209 = One Button Dialog(message="Data File Not Found") -> ()  [unwired: 1 in, 1 out]
                  }
                }
                n210 = case shown="Faux" w388 {
                  frame False {
                    n211 = One Button Dialog(message="X Parameter not found. Using Column \"0\".") -> ()  [unwired: 1 in, 1 out]
                  }
                  frame True {
                  }
                }
              }
              frame "Opentxt" {
                n212 = property class="Arbre (strict)"(reference=w501, error in=w500) -> (error out=w490:errorcluster, "Active Item Tag"=w489:string)  [unwired: 1 out]
                n213 = Scan From String(format string="%4s-%2s-%2s_S%d_Sc%d_%d_f%d" ("chaîne de format"), input string=w489, error in=w490, default 5=i64 0 ("valeur par défaut 5")) -> (error out=w491:errorcluster, output 6=w492:i32, output 7=w494:i32)  [unwired: 12 in, 2 out]
                n214 = case shown="Pas d'erreur" w491 {
                  selector: w491 -> [w513 _]
                  tunnel: w494 -> [w515 _]
                  tunnel: [w515 w517] -> w493
                  tunnel: [w514 w516] -> _
                  tunnel: w492 -> [w514 _]
                  tunnel: [w513 w518] -> w483
                  tunnel: w490 -> [_ w519]
                  tunnel: w489 -> [_ w522]
                  tunnel: "%4s-%2s-%2s_S%d_Sc%d_%d_%d_f%d" ("chaîne de format") -> [_ w521]
                  frame No Error {
                  }
                  frame Error {
                    n215 = Scan From String(format string=w521, input string=w522, error in=w519, default 5=i64 0 ("valeur par défaut 5")) -> (error out=w518:errorcluster, output 7=w516:i32, output 8=w517:i32)  [unwired: 14 in, 2 out]
                  }
                }
                n216 = local read "FilesPath"() -> (w495:path[])
                n217 = Index Array(array=w495, index=w493) -> (element=w487:path)
                n218 = Strip Path(path=w487) -> (stripped path=w477:path, name=w486:string)
                n219 = Search and Replace String(input string=w486, search string="Header" ("sous-chaîne (\"\")"), replace string="Data" ("chaîne de remplacement (\"\")"), error in=w483) -> (result string=w481:string, error out=w482:errorcluster)  [unwired: 4 in, 2 out]
                n220 = Search and Replace String(input string=w481, search string=".dat" ("chaîne recherchée"), replace string=".txt" ("chaîne de remplacement (\"\")"), error in=w482) -> (result string=w478:string, error out=w476:errorcluster)  [unwired: 4 in, 2 out]
                n221 = Build Path(base path=w477, name or relative path=w478) -> (appended path=w474:path)
                n222 = case shown="Pas d'erreur" w476 {
                  selector: w476 -> [w503 w510]
                  tunnel: [w502 w511] -> w475
                  tunnel: w474 -> [w504 _]
                  frame No Error {
                    n223 = Path To String(path=w504) -> (string=w506:string)
                    n224 = Concatenate Strings("notepad" ("command line"), " " ("string"), w506) -> (w505:string)
                    n225 = call <vilib>:"System Exec.vi"("wait until completion? (T)"=FALSE, "error in (no error)"=w503, "command line"=w505) -> ("error out"=w502:errorcluster)  [unwired: 5 in, 3 out]
                  }
                  frame Error {
                    n226 = call <vilib>:"Clear Errors.vi"("error in (no error)"=w510) -> ("error out"=w511:errorcluster)  [unwired: 5 in, 1 out]
                    n227 = One Button Dialog(message="Data File Not Found") -> ()  [unwired: 1 in, 1 out]
                  }
                }
              }
              frame "Delete File" {
                n228 = property class="Arbre (strict)"(reference=w551, error in=w550) -> (error out=w540:errorcluster, "Active Item Tag"=w539:string)  [unwired: 1 out]
                n229 = Scan From String(format string="%4s-%2s-%2s_S%d_Sc%d_%d_f%d" ("chaîne de format"), input string=w539, error in=w540, default 5=i64 0 ("valeur par défaut 5")) -> (error out=w541:errorcluster, output 6=w542:i32, output 7=w544:i32)  [unwired: 12 in, 2 out]
                n230 = case shown="Pas d'erreur" w541 {
                  selector: w541 -> [w572 _]
                  tunnel: w544 -> [w574 _]
                  tunnel: [w574 w576] -> w543
                  tunnel: [w573 w575] -> _
                  tunnel: w542 -> [w573 _]
                  tunnel: [w572 w577] -> w534
                  tunnel: w540 -> [_ w578]
                  tunnel: w539 -> [_ w581]
                  tunnel: "%4s-%2s-%2s_S%d_Sc%d_%d_%d_f%d" ("chaîne de format") -> [_ w580]
                  frame No Error {
                  }
                  frame Error {
                    n231 = Scan From String(format string=w580, input string=w581, error in=w578, default 5=i64 0 ("valeur par défaut 5")) -> (error out=w577:errorcluster, output 7=w575:i32, output 8=w576:i32)  [unwired: 14 in, 2 out]
                  }
                }
                n232 = local read "FilesPath"() -> (w545:path[])
                n233 = Index Array(array=w545, index=w543) -> (element=w525:path)
                n234 = Strip Path(path=w525) -> (stripped path=w528:path, name=w537:string)
                n235 = Search and Replace String(input string=w537, search string="Header" ("sous-chaîne (\"\")"), replace string="Data" ("chaîne de remplacement (\"\")"), error in=w534) -> (result string=w532:string, error out=w533:errorcluster)  [unwired: 4 in, 2 out]
                n236 = Search and Replace String(input string=w532, search string=".dat" ("chaîne recherchée"), replace string=".txt" ("chaîne de remplacement (\"\")"), error in=w533) -> (result string=w529:string, error out=w526:errorcluster)  [unwired: 4 in, 2 out]
                n237 = Build Path(base path=w528, name or relative path=w529) -> (appended path=w527:path)
                n238 = case shown="Pas d'erreur" w526 {
                  selector: w526 -> [w555 w569]
                  tunnel: [w553 w570] -> w524
                  tunnel: w527 -> [w554 _]
                  tunnel: w525 -> [w556 _]
                  tunnel: w523 -> [w552 _]
                  frame No Error {
                    n239 = Two Button Dialog(message="This will delete the selected curve data file permanently with all other curves it includes. Proceed?") -> (T button?=w557:bool)  [unwired: 2 in]
                    n240 = case shown="Vrai" w557 {
                      tunnel: w555 -> [w559 w567]
                      tunnel: w556 -> [_ w566]
                      tunnel: w554 -> [_ w568]
                      tunnel: [w559 w561] -> w553
                      tunnel: w552 -> [_ w560]
                      frame False {
                      }
                      frame True {
                        n241 = Delete(path (use dialog)=w568, error in=w567) -> (error out=w564:errorcluster)  [unwired: 3 in, 2 out]
                        n242 = Delete(path (use dialog)=w566, error in=w567) -> (error out=w565:errorcluster)  [unwired: 3 in, 2 out]
                        n243 = Merge Errors(w564, w565) -> (w562:errorcluster)
                        n244 = Enqueue Element(queue=w560, element=BrowseDataStates."LoadTree" ("Énum"), error in (no error)=w562) -> (error out=w561:errorcluster)  [unwired: 1 in, 2 out]
                      }
                    }
                  }
                  frame Error {
                    n245 = call <vilib>:"Clear Errors.vi"("error in (no error)"=w569) -> ("error out"=w570:errorcluster)  [unwired: 5 in, 1 out]
                    n246 = One Button Dialog(message="Data File Not Found") -> ()  [unwired: 1 in, 1 out]
                  }
                }
              }
              frame "OpenCurve" {
                n247 = local read "Curve Preview"() -> (w595:cluster{"X Array":dbl[], "Y Array":dbl[]})
                n248 = Unbundle(w595) -> ("X Array"=w592:dbl[], "Y Array"=w591:dbl[])
                n249 = Array Size(array=w592) -> (size(s)=w593:i32)
                n250 = Greater Than 0?(x=w593) -> (x > 0?=w594:bool)
                n251 = case shown="Vrai" w594 {
                  tunnel: w598 -> [w600 w608]
                  tunnel: [w600 w607] -> w584
                  tunnel: w597 -> [w599 w606]
                  tunnel: [w599 w605] -> w583
                  tunnel: w592 -> [_ w604]
                  tunnel: w591 -> [_ w603]
                  frame False {
                  }
                  frame True {
                    n252 = local read "CurveName"() -> (w602:string)
                    n253 = local read "VarPar"() -> (w601:string)
                    n254 = call "AddCurve.vi"("VarPar"=w601, "CurveName"=w602, "error in"=w606, "Y Array"=w603, "X Array"=w604, "InterfaceIn"=w608) -> ("error out"=w605:errorcluster, "InterfaceOut"=w607:refnum<class "Interface.lvclass">)  [unwired: 4 in]
                  }
                }
                n255 = Bundle By Name(cluster=cluster{"Message":string, "Data":variant, i32} {"Message"="UpdateItf", "Data"=variant, 0} ("élément"), "Data"=w584) -> (w587:cluster{"Message":string, "Data":variant, i32})
                n256 = Enqueue Element(queue=w585, element=w587, error in (no error)=w583) -> (queue out=w590:refnum<queue>, error out=w589:errorcluster)  [unwired: 1 in, 1 out]
                n257 = Generate User Event(user event=w586, event data cluster=w590, error in=w589) -> (error out=w582:errorcluster)  [unwired: 1 in, 1 out]
              }
              frame "Open2D" {
                w614 = cluster{"Message":string, "Data":variant, i32} {"Message"="", "Data"=variant, 0} ("élément")
                n258 = local read "Data path"() -> (w640:path)
                n259 = call "AddNew2DGraph.vi"("error in (no error)"=w639, "DataFileName"=w640, "Interface en entrée"=w642) -> ("error out"=w638:errorcluster, "Graph"=w620:refnum<vi>, "Interface en sortie"=w641:refnum<class "Interface.lvclass">, "2DGraphQRef"=w621:refnum<queue>)  [unwired: 4 in, 1 out]
                n260 = local read "Y Parameters"() -> (w644:u16)
                n261 = local read "X Parameters"() -> (w645:u16)
                n262 = local read "Header path"() -> (w643:path)
                n263 = call "DataRead2D.vi"("Chemin Header"=w643, "chemin Data"=w640, "ScanlistIndex"=w644, "error in"=w638, "XVarParIndex"=w645) -> ("2D_Data"=w612:dbl[][], "VarParx"=w624:string, "VarPary"=w625:string, "X Array"=w618:dbl[], "Y Array 2D"=w622:dbl[], "CurveName"=w623:string, "error out"=w619:errorcluster)  [unwired: 1 in, 3 out]
                n264 = Array Size(array=w618) -> (size(s)=w617:i32)
                n265 = Array Size(array=w622) -> (size(s)=w637:i32)
                n266 = Build Array(w617, w637) -> (w634:i32[])
                n267 = Index Array(array=w618) -> (element #1=w628:dbl, element #2=w629:dbl)  [unwired: 2 in]
                n268 = Index Array(array=w622) -> (element #1=w626:dbl, element #2=w627:dbl)  [unwired: 2 in]
                n269 = To Variant(anything=w634) -> (Variant=w633:variant)
                n270 = Subtract(x=w629, y=w628) -> (x-y=w631:dbl)
                n271 = Subtract(x=w627, y=w626) -> (x-y=w630:dbl)
                n272 = Bundle(cluster=w614, "Message"="InitGraph", "Data"=w633) -> (w636:cluster{"Message":string, "Data":variant, i32})  [unwired: 1 in]
                n273 = Enqueue Element(queue=w621, element=w636, error in (no error)=w619) -> (queue out=w616:refnum<queue>, error out=w632:errorcluster)  [unwired: 1 in, 1 out]
                n274 = property class="GraphInt"(reference=w620, error in=w632, "XScale.Multiplier"=w631, "XScale.Offset"=w628, "YScale.Multiplier"=w630, "YScale.Offset"=w626, "XScale.NameLbl.Text"=w624, "YScale.NameLbl.Text"=w625, "ZScale.NameLbl.Text"=w623) -> (error out=w615:errorcluster)  [unwired: 1 out]
                n275 = To Variant(anything=w612) -> (Variant=w611:variant)
                n276 = Bundle(cluster=w614, "Message"="UpdateWhole", "Data"=w611) -> (w610:cluster{"Message":string, "Data":variant, i32})  [unwired: 1 in]
                n277 = Enqueue Element(queue=w616, element=w610, error in (no error)=w615) -> (error out=w609:errorcluster)  [unwired: 1 in, 2 out]
              }
              frame "Stop", Default {
              }
            }
          }
          frame Error {
            n278 = call <vilib>:"Clear Errors.vi"("error in (no error)"=w654) -> ("error out"=w651:errorcluster)  [unwired: 5 in, 1 out]
          }
        }
      }
      n279 = Merge Errors(w16, w15) -> (w14:errorcluster)
      n280 = Release Queue(queue=w21, error in (no error)=w14) -> (error out=w23:errorcluster)  [unwired: 1 in, 2 out]
    }
    frame Error {
    }
  }
  "sortie d'erreur" <- w6
  "Interface en sortie" <- w4
